vi "Build_database_info.vi"(7 "Collection Info Array":T2[](array[typedef]), 9 "Chemical":string, 10 "RingText.Text":string, 11 "New Date Name":string) -> (3 "Data to add":T1)   [LabVIEW 2019]
uses:
  Type defs/FileAcq_v1_Ctrl.ctl
  Type defs/Database_control.ctl
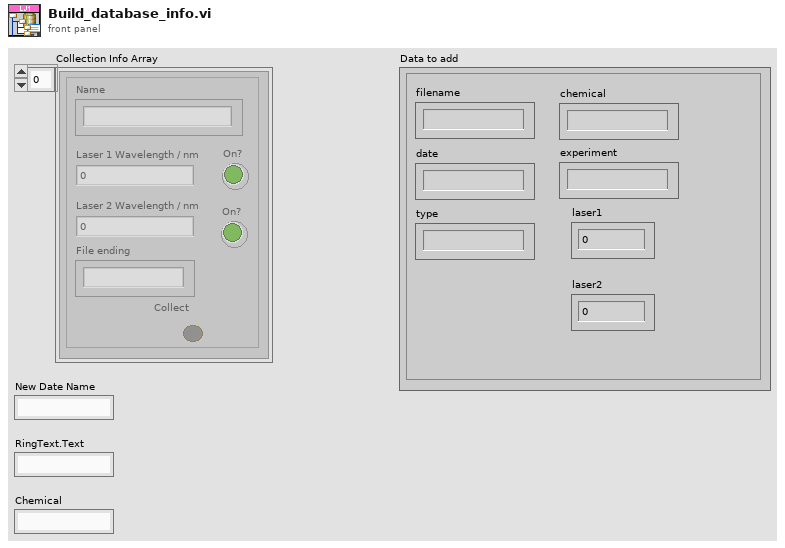
[diagram p1: front panel]
types:
  T1 = typedef "Database_control.ctl" = cluster{"filename":string, "date":string, "type":string, "chemical":string, "experiment":string, "laser1":dbl, "laser2":dbl}
  T2 = typedef "FileAcq_v1_Ctrl.ctl" = cluster{"Type":string, "LaserWave1":dbl, "Shutter1":bool, "LaserWave2":dbl, "Shutter2":bool, "FileEnd":string, "Collect":bool}
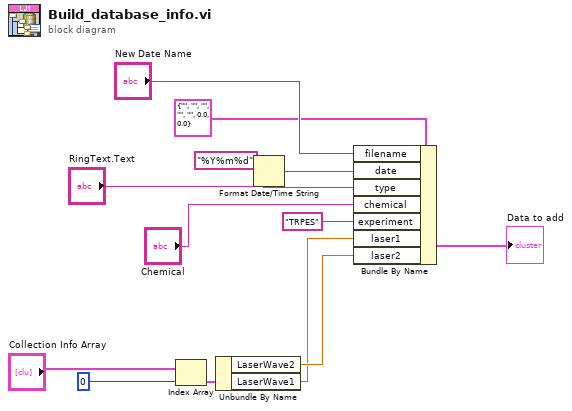
[diagram p0: block diagram]
diagram:
  n1 = Index Array(array="Collection Info Array", index=0) -> (element=w8:T2)
  n2 = Unbundle By Name(w8) -> ("LaserWave2"=w10:dbl, "LaserWave1"=w9:dbl)
  n3 = Format Date/Time String(time format string (%c)="%Y%m%d") -> (date/time string=w4:string)  [unwired: 2 in]
  n4 = Bundle By Name(cluster=T1 {"filename"="", "date"="", "type"="", "chemical"="", "experiment"="", "laser1"=0.0, "laser2"=0.0} ("Data to add"), "filename"="New Date Name", "date"=w4, "type"="RingText.Text", "chemical"="Chemical", "experiment"="TRPES", "laser1"=w9, "laser2"=w10) -> (→"Data to add":T1)
